vi "ServoTempReadIn.vi"(10 "Command":string="UU\u0001\u0005\u001cþÿà") -> (1 "Temp":u8 max=240 step=1, 2 "ID":u8=1)   [LabVIEW 2013]
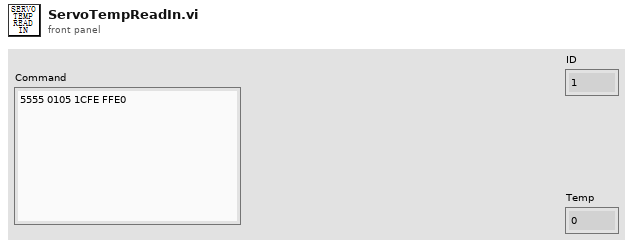
[diagram p1: front panel]
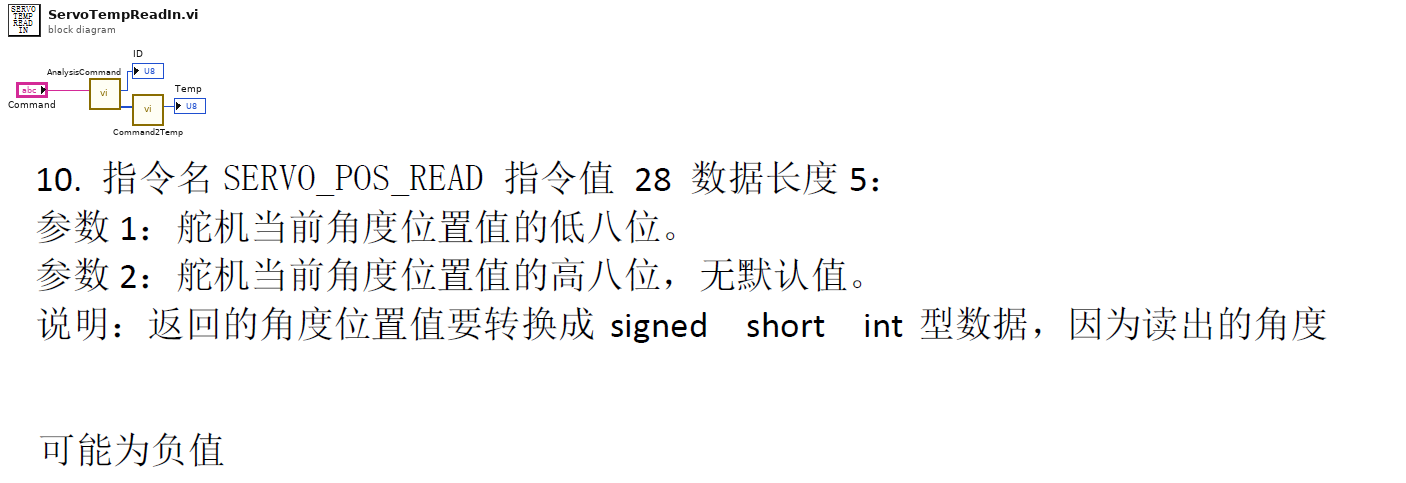
[diagram p0: block diagram]
diagram:
  n1 = call "AnalysisCommand.vi"("Command"="Command") -> ("DataOut"=w2:u8[], "ID"=→"ID":u8)  [unwired: 8 in, 1 out]
  n2 = call "Command2Temp.vi"("DataIn"=w2) -> ("Temp"=→"Temp":u8)  [unwired: 10 in]
